vi "Write ID.vi"(8 "error in":errorcluster, 10 "ID":string, 11 "DAQ Device in":refnum<class "DAQ Device.lvclass">) -> (0 "error out":errorcluster, 3 "DAQ Device out":refnum<class "DAQ Device.lvclass">)   [LabVIEW 2014, in "DAQ Device.lvclass"]
uses:
  DAQ Device.lvclass
  DAQ Device.lvclass/DAQ Device.ctl
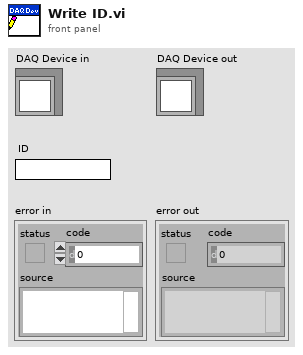
[diagram p1: front panel]
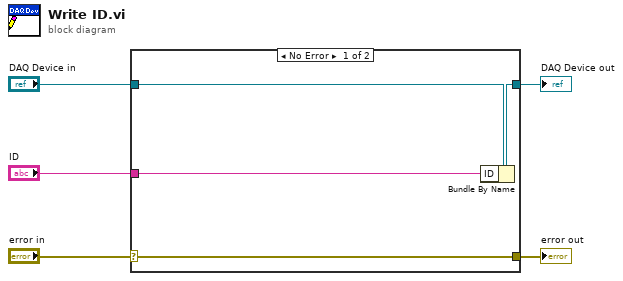
[diagram p0: block diagram]
diagram:
  n1 = case shown="No Error" "error in" {
    selector: "error in" -> [w9 w10]
    tunnel: [w9 w10] -> w4
    tunnel: [w7 w11] -> w2
    tunnel: "DAQ Device in" -> [w8 w11]
    tunnel: "ID" -> [w6 _]
    frame No Error {
      n2 = Bundle By Name(cluster=w8, "ID"=w6) -> (w7:refnum<class "DAQ Device.lvclass">)
    }
    frame Error {
    }
  }
  "error out" <- w4
  "DAQ Device out" <- w2
